vi "StartVLCPlayer.vi"(8 "error in":errorcluster, 9 "VLC executable path":path=path "C:/Program Files (x86)/VideoLAN/VLC/vlc.exe", 10 "VLC Port":u16=65123, 11 "VLC IP address":string="127.0.0.1") -> (0 "error out":errorcluster)   [LabVIEW 2015]
doc: "Low level VI to start a VLC player process. Generally don't use this, use \"OpenVLCPLayer\" instead."
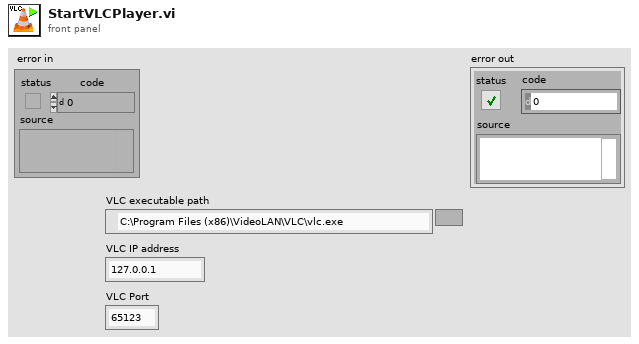
[diagram p1: front panel]
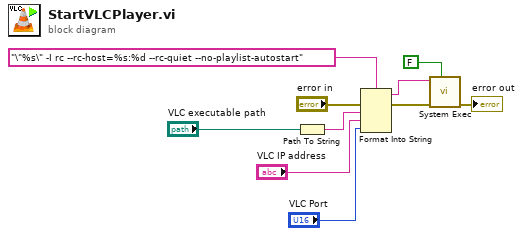
[diagram p0: block diagram]
diagram:
  n1 = Path To String(path="VLC executable path") -> (string=w9:string)
  n2 = Format Into String(format string="\"%s\" -I rc --rc-host=%s:%d --rc-quiet --no-playlist-autostart", error in="error in", w9, "VLC IP address", "VLC Port") -> (resulting string=w10:string, error out=w2:errorcluster)  [unwired: 1 in]
  n3 = call <vilib>:"System Exec.vi"("wait until completion? (T)"=FALSE, "error in (no error)"=w2, "command line"=w10) -> ("error out"=→"error out":errorcluster)  [unwired: 5 in, 3 out]
